vi "Abort_VI.vi"(8 "error in (no error)":errorcluster, 9 "Message_command_in":T1, 10 "Command Queue in":T2) -> (0 "error out":errorcluster, 1 "Message_command out":T1, 2 "Command Queue out":T2, 11 "machine name (\"\":  open local reference)":string)   [LabVIEW 2019]
uses:
  Command_Queue.ctl
  Command_Message.ctl
panel:
  in  "port":u16=3374
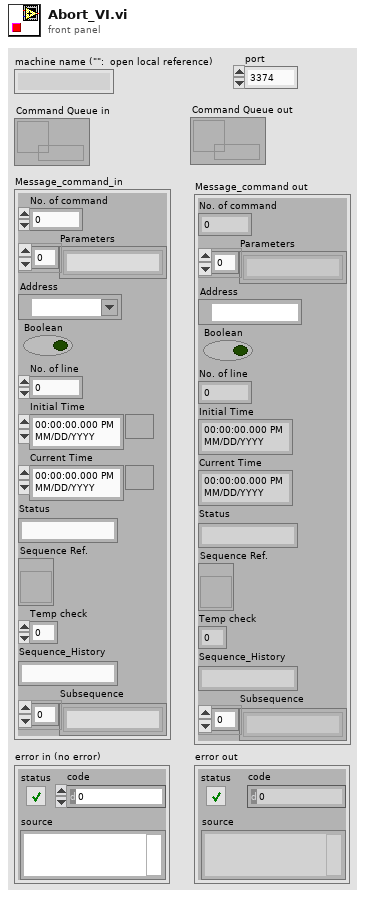
[diagram p1: front panel]
types:
  T1 = typedef "Command_Message.ctl" = cluster{"No. of command":i32, "Parameters":string[], "Address":refnum<visa-resource-name>, "Boolean":bool, "No. of line":i32, "Initial Time":timestamp, "Current Time":timestamp, "Status":string, "Sequence Ref.":refnum<vi>, "Temp check":i32, "Sequence_History":string, "Subsequence":string[]}
  T2 = typedef "Command_Queue.ctl" = refnum<queue>
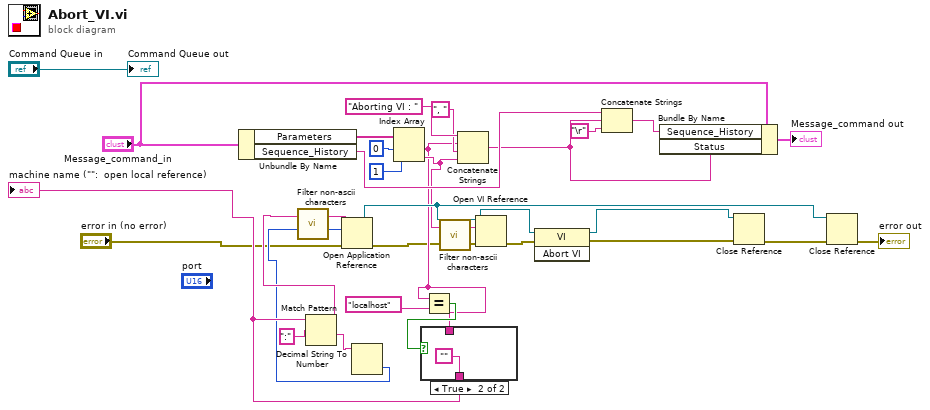
[diagram p0: block diagram]
diagram:
  n1 = Unbundle By Name("Message_command_in") -> ("Parameters"=w31:string[], "Sequence_History"=w23:string)
  n2 = Index Array(array=w31, index #1=0 ("index"), index #2=1 ("index")) -> (element #1=w8:string, element #2=w14:string)
  n3 = Equal?(x=w8, y="localhost") -> (x = y?=w16:bool)
  n4 = case shown="True" w16 {
    tunnel: [w33 ""] -> w11
    tunnel: w8 -> [w33 _]
    frame False {
    }
    frame True {
    }
  }
  "machine name (\"\":  open local reference)" <- w11
  n5 = Match Pattern(string=w11, regular expression=":") -> (before substring=w10:string, after substring=w12:string)  [unwired: 1 in, 2 out]
  n6 = call "Filter non-ascii characters.vi"(2:w10) -> ("output"=w2:string)  [unwired: 1 in]
  n7 = Decimal String To Number(string=w12) -> (number=w9:i32)  [unwired: 2 in, 1 out]
  n8 = Open Application Reference(8:"error in (no error)", 10:w9, 11:w2) -> (0:w6:errorcluster, 3:w27:refnum<vi>)  [unwired: 1 in]
  n9 = call "Filter non-ascii characters.vi"(2:w14) -> ("output"=w1:string)  [unwired: 1 in]
  n10 = Concatenate Strings("Aborting VI : " ("string"), w8, ", " ("string"), w14) -> (w20:string)
  n11 = Open VI Reference(application reference (local)=w27, vi path=w1, error in (no error)=w6) -> (vi reference=w29:refnum<vi>, error out=w5:errorcluster)  [unwired: 3 in]
  n12 = invoke class="VI" method="Abort VI"(reference=w29, error in=w5) -> (reference out=w28:refnum<vi>, error out=w4:errorcluster)  [unwired: 1 in, 1 out]
  n13 = Concatenate Strings(w23, w20, "\r") -> (w21:string)
  n14 = Bundle By Name(cluster="Message_command_in", "Sequence_History"=w21, "Status"=w20) -> (→"Message_command out":T1)
  n15 = Close Reference(reference=w28, error in (no error)=w4) -> (error out=w3:errorcluster)
  n16 = Close Reference(reference=w27, error in (no error)=w3) -> (error out=→"error out":errorcluster)
  "Command Queue out" <- "Command Queue in"
